vi "Flush Queue.vi"(8 "error in (no error)":errorcluster, 10 "Data Type":T12, 11 "Sift Client in":refnum<class "Sift Client.lvclass">) -> (0 "error out":errorcluster, 3 "Sift Client out":refnum<class "Sift Client.lvclass">)   [LabVIEW 2024, in "Sift Client.lvlib" / "Sift Client.lvclass"]
uses:
  Sift Client.lvclass
  Generate Sift Protos/SiftProxy_client/RPC Messages/sift_proxy_v1_ChannelDataType.ctl
  Generate Sift Protos/SiftProxy_client/RPC Messages/sift_proxy_v1_IngestDataStreamDoubleRequest.ctl
  Generate Sift Protos/SiftProxy_client/RPC Messages/google_protobuf_Timestamp.ctl
  Generate Sift Protos/SiftProxy_client/RPC Messages/sift_proxy_v1_IngestDataStreamStringRequest.ctl
  Generate Sift Protos/SiftProxy_client/RPC Messages/sift_proxy_v1_IngestDataStreamEnumRequest.ctl
  Generate Sift Protos/SiftProxy_client/RPC Messages/sift_proxy_v1_IngestDataStreamBytesRequest.ctl
  Generate Sift Protos/SiftProxy_client/RPC Messages/sift_proxy_v1_IngestDataStreamBoolRequest.ctl
  Generate Sift Protos/SiftProxy_client/RPC Messages/sift_proxy_v1_IngestDataStreamFloatRequest.ctl
  Generate Sift Protos/SiftProxy_client/RPC Messages/sift_proxy_v1_IngestDataStreamInt32Request.ctl
  Generate Sift Protos/SiftProxy_client/RPC Messages/sift_proxy_v1_IngestDataStreamUInt32Request.ctl
  Generate Sift Protos/SiftProxy_client/RPC Messages/sift_proxy_v1_IngestDataStreamInt64Request.ctl
  Generate Sift Protos/SiftProxy_client/RPC Messages/sift_proxy_v1_IngestDataStreamUInt64Request.ctl
  Sift Client.lvclass/Sift Client.ctl
  Generate Sift Protos/SiftProxy_client/SiftProxy_client.lvlib
panel:
  in  "sift_proxy_v1_IngestDataStreamUInt64Request":T1
  in  "sift_proxy_v1_IngestDataStreamInt64Request":T3
  in  "sift_proxy_v1_IngestDataStreamUInt32Request":T4
  in  "sift_proxy_v1_IngestDataStreamInt32Request":T5
  in  "sift_proxy_v1_IngestDataStreamFloatRequest":T6
  in  "sift_proxy_v1_IngestDataStreamBoolRequest":T7
  in  "sift_proxy_v1_IngestDataStreamBytesRequest":T8
  in  "sift_proxy_v1_IngestDataStreamEnumRequest":T9
  in  "sift_proxy_v1_IngestDataStreamStringRequest":T10
  in  "sift_proxy_v1_IngestDataStreamDoubleRequest":T11
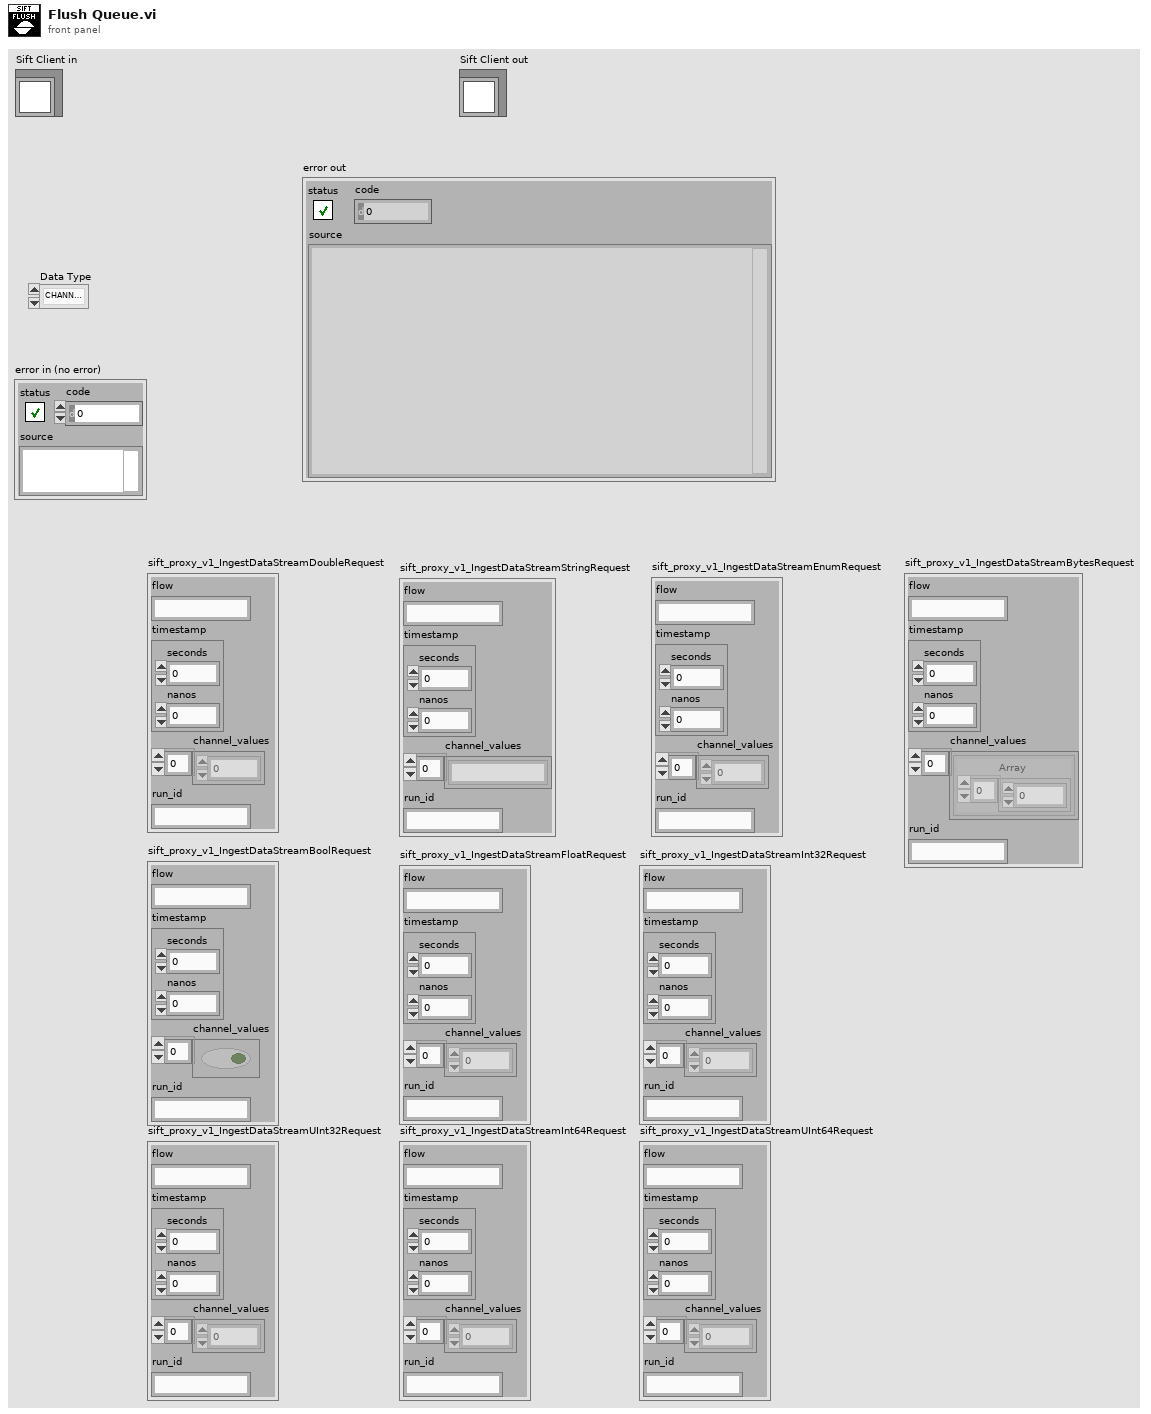
[diagram p1: front panel]
types:
  T1 = typedef "SiftProxy_client.lvlib/sift_proxy_v1_IngestDataStreamUInt64Request.ctl" = cluster{"flow":string, "timestamp":T2, "channel_values":u64[], "run_id":string}
  T2 = typedef "SiftProxy_client.lvlib/google_protobuf_Timestamp.ctl" = cluster{"seconds":i64, "nanos":i32}
  T3 = typedef "SiftProxy_client.lvlib/sift_proxy_v1_IngestDataStreamInt64Request.ctl" = cluster{"flow":string, "timestamp":T2, "channel_values":i64[], "run_id":string}
  T4 = typedef "SiftProxy_client.lvlib/sift_proxy_v1_IngestDataStreamUInt32Request.ctl" = cluster{"flow":string, "timestamp":T2, "channel_values":u32[], "run_id":string}
  T5 = typedef "SiftProxy_client.lvlib/sift_proxy_v1_IngestDataStreamInt32Request.ctl" = cluster{"flow":string, "timestamp":T2, "channel_values":i32[], "run_id":string}
  T6 = typedef "SiftProxy_client.lvlib/sift_proxy_v1_IngestDataStreamFloatRequest.ctl" = cluster{"flow":string, "timestamp":T2, "channel_values":sgl[], "run_id":string}
  T7 = typedef "SiftProxy_client.lvlib/sift_proxy_v1_IngestDataStreamBoolRequest.ctl" = cluster{"flow":string, "timestamp":T2, "channel_values":bool[], "run_id":string}
  T8 = typedef "SiftProxy_client.lvlib/sift_proxy_v1_IngestDataStreamBytesRequest.ctl" = cluster{"flow":string, "timestamp":T2, "channel_values":cluster{"Array":u8[]}[], "run_id":string}
  T9 = typedef "SiftProxy_client.lvlib/sift_proxy_v1_IngestDataStreamEnumRequest.ctl" = cluster{"flow":string, "timestamp":T2, "channel_values":u32[], "run_id":string}
  T10 = typedef "SiftProxy_client.lvlib/sift_proxy_v1_IngestDataStreamStringRequest.ctl" = cluster{"flow":string, "timestamp":T2, "channel_values":string[], "run_id":string}
  T11 = typedef "SiftProxy_client.lvlib/sift_proxy_v1_IngestDataStreamDoubleRequest.ctl" = cluster{"flow":string, "timestamp":T2, "channel_values":dbl[], "run_id":string}
  T12 = typedef "SiftProxy_client.lvlib/sift_proxy_v1_ChannelDataType.ctl" = enum32{"CHANNEL_DATA_TYPE_UNSPECIFIED", "CHANNEL_DATA_TYPE_DOUBLE", "CHANNEL_DATA_TYPE_STRING", "CHANNEL_DATA_TYPE_ENUM", "CHANNEL_DATA_TYPE_BIT_FIELD", "CHANNEL_DATA_TYPE_BOOL", "CHANNEL_DATA_TYPE_FLOAT", "CHANNEL_DATA_TYPE_INT_32", "CHANNEL_DATA_TYPE_UINT_32", "CHANNEL_DATA_TYPE_INT_64", "CHANNEL_DATA_TYPE_UINT_64"}
  T13 = typedef "Sift Client.lvlib/Double Sample.ctl" = cluster{"Values":dbl[], "Timestamp":T2, "Flow Name":string}
  T14 = typedef "grpc-lvsupport-release.lvlib/grpcId.ctl" = u64
  T15 = typedef "Sift Client.lvlib/String Sample.ctl" = cluster{"Values":string[], "Timestamp":T2, "Flow Name":string}
  T16 = typedef "Sift Client.lvlib/Enum Sample.ctl" = cluster{"Values":u32[], "Timestamp":T2, "Flow Name":string}
  T17 = typedef "Sift Client.lvlib/Bitfield Sample.ctl" = cluster{"Timestamp":T2, "Values":cluster{"Array":u8[]}[], "Flow Name":string}
  T18 = typedef "Sift Client.lvlib/Bool Sample.ctl" = cluster{"Values":bool[], "Timestamp":T2, "Flow Name":string}
  T19 = typedef "Sift Client.lvlib/Float Sample.ctl" = cluster{"Values":sgl[], "Timestamp":T2, "Flow Name":string}
  T20 = typedef "Sift Client.lvlib/Int32 Sample.ctl" = cluster{"Values":i32[], "Timestamp":T2, "Flow Name":string}
  T21 = typedef "Sift Client.lvlib/Uint32 Sample.ctl" = cluster{"Values":u32[], "Timestamp":T2, "Flow Name":string}
  T22 = typedef "Sift Client.lvlib/Int64 Sample.ctl" = cluster{"Values":i64[], "Timestamp":T2, "Flow Name":string}
  T23 = typedef "Sift Client.lvlib/Uint64 Sample.ctl" = cluster{"Values":u64[], "Timestamp":T2, "Flow Name":string}
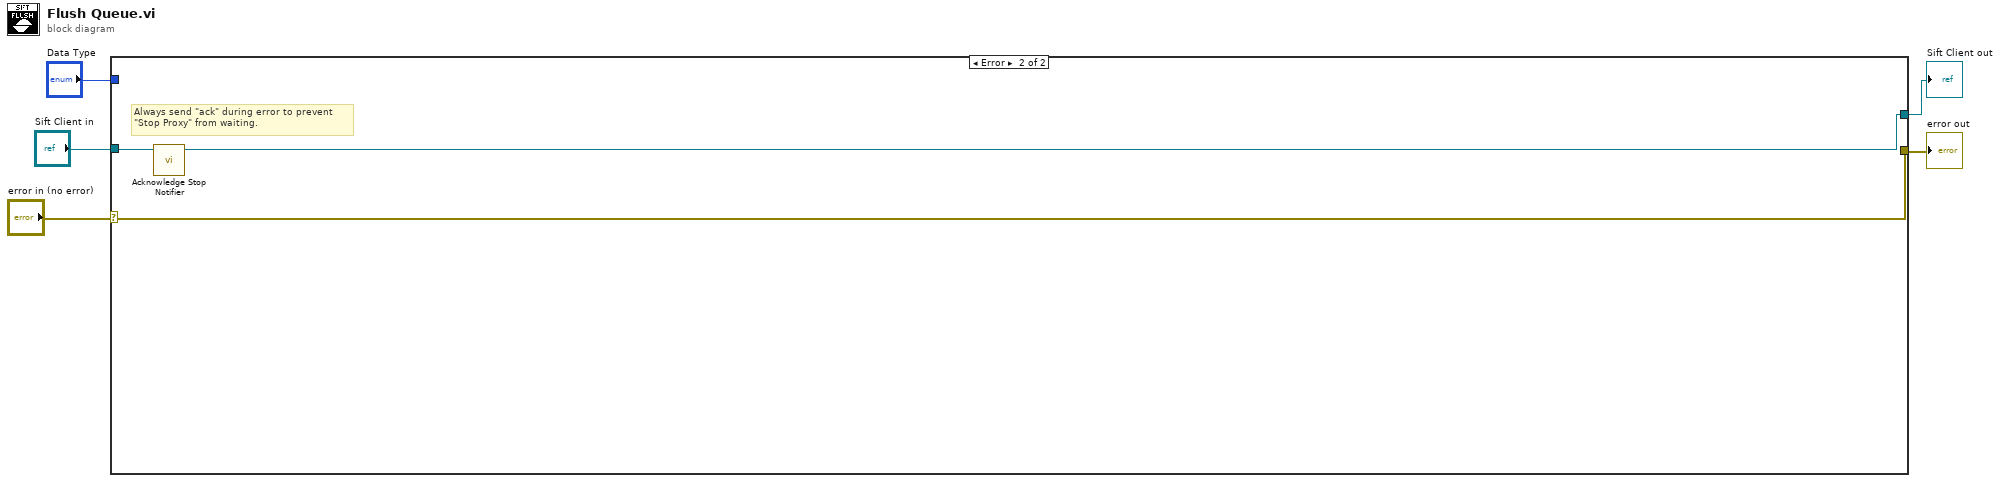
[diagram p0: block diagram]
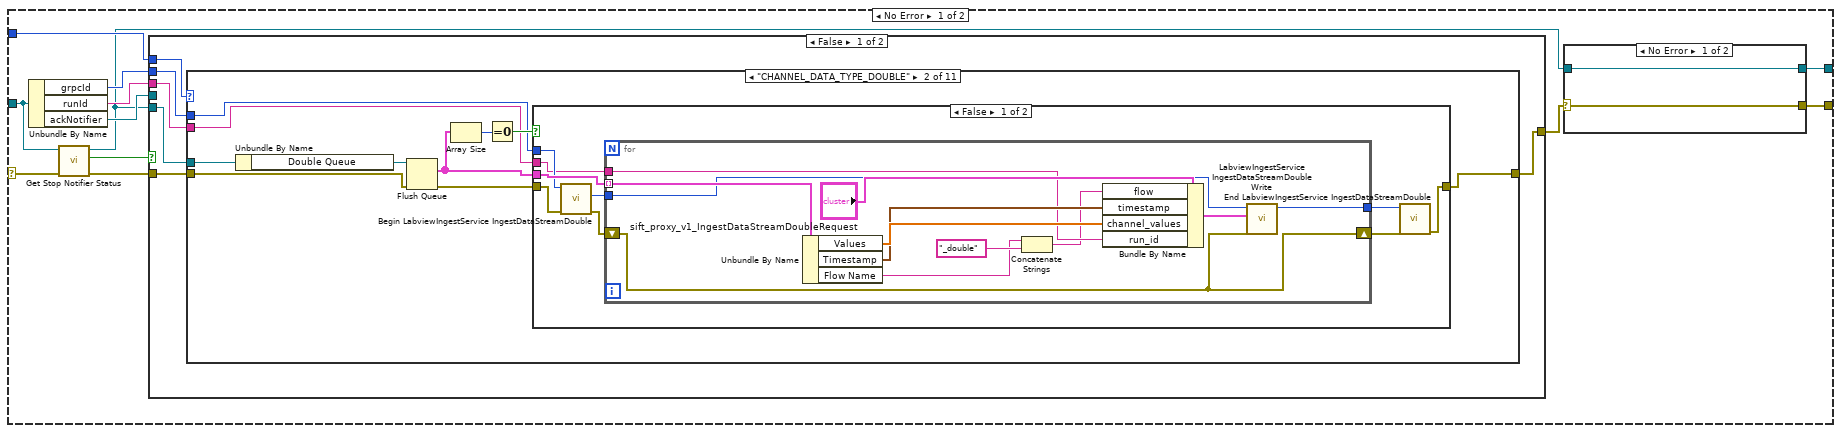
[diagram p2: hidden frame]
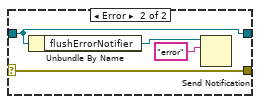
[diagram p3: hidden frame]
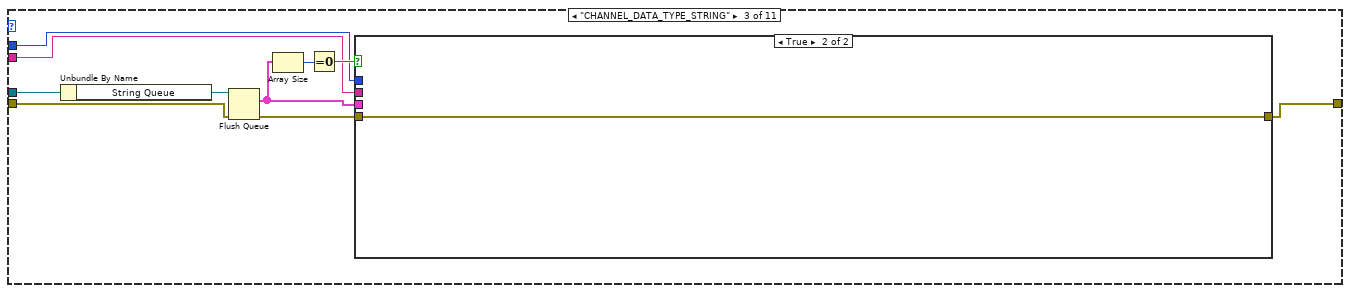
[diagram p6: hidden frame]
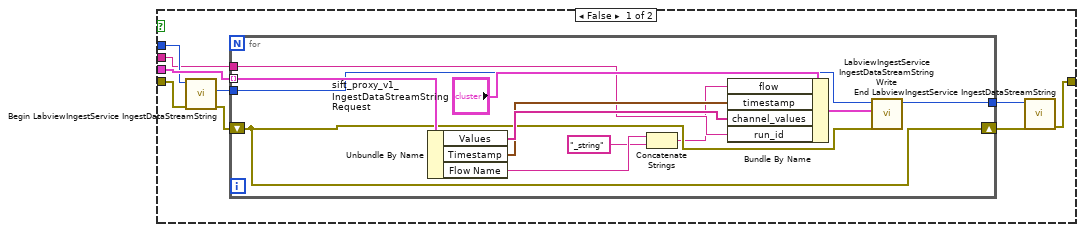
[diagram p7: hidden frame]
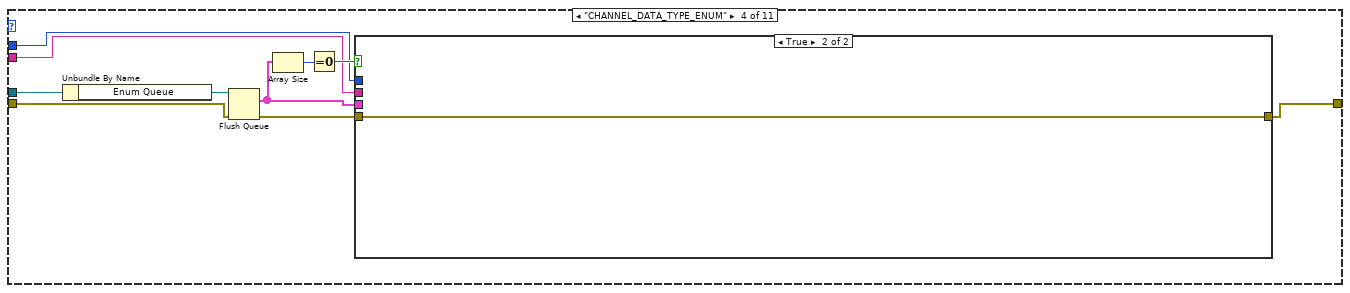
[diagram p8: hidden frame]
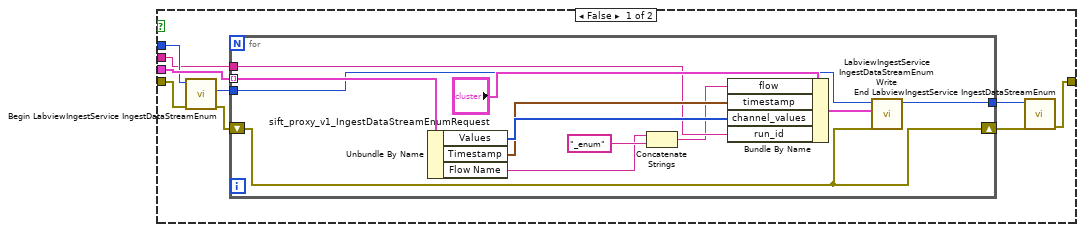
[diagram p9: hidden frame]
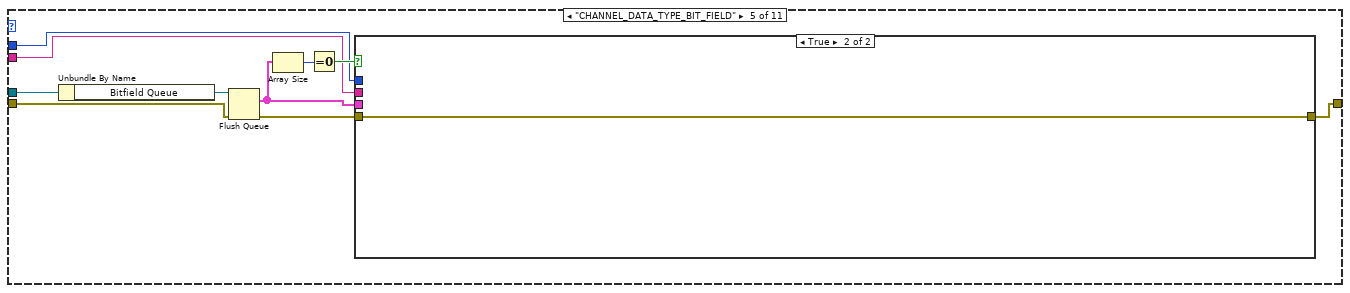
[diagram p10: hidden frame]
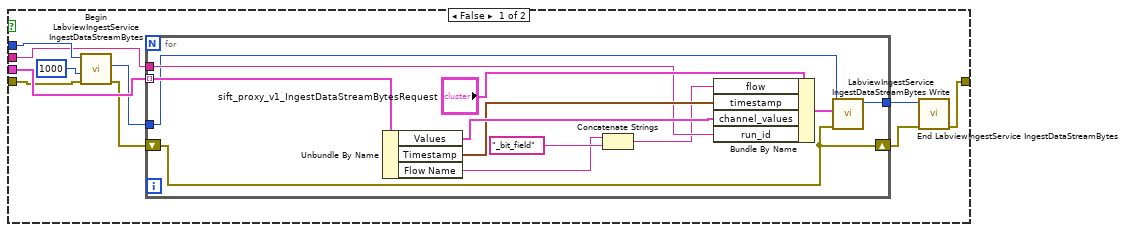
[diagram p11: hidden frame]
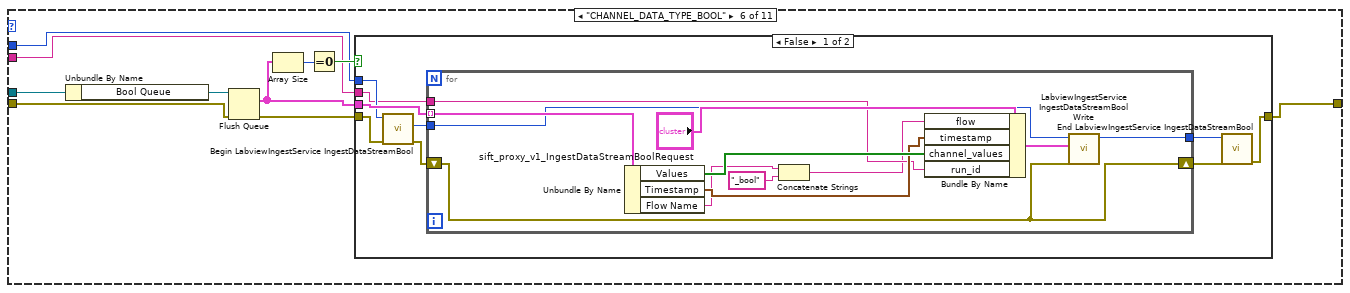
[diagram p12: hidden frame]
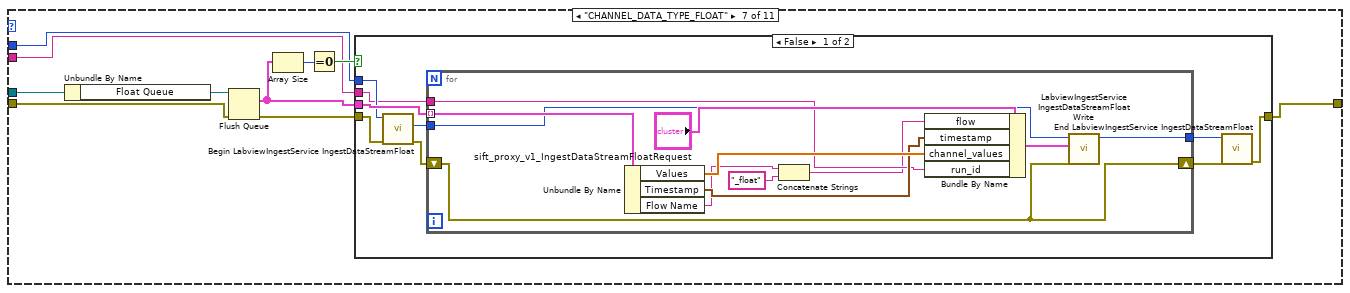
[diagram p14: hidden frame]
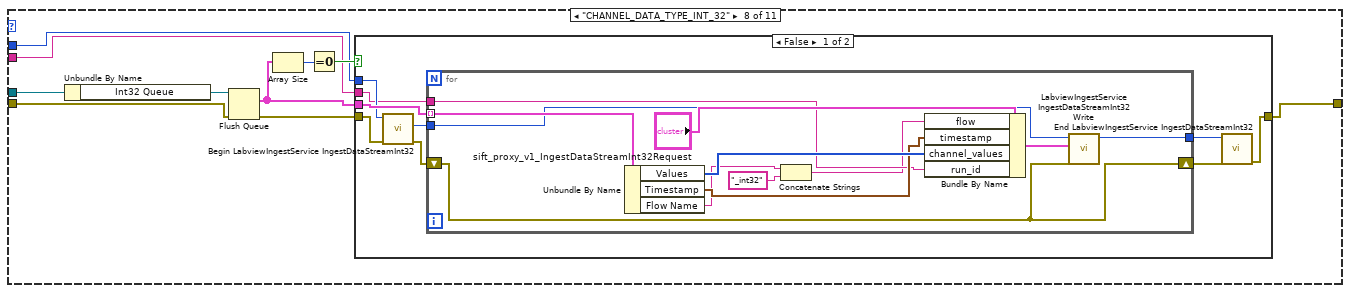
[diagram p16: hidden frame]
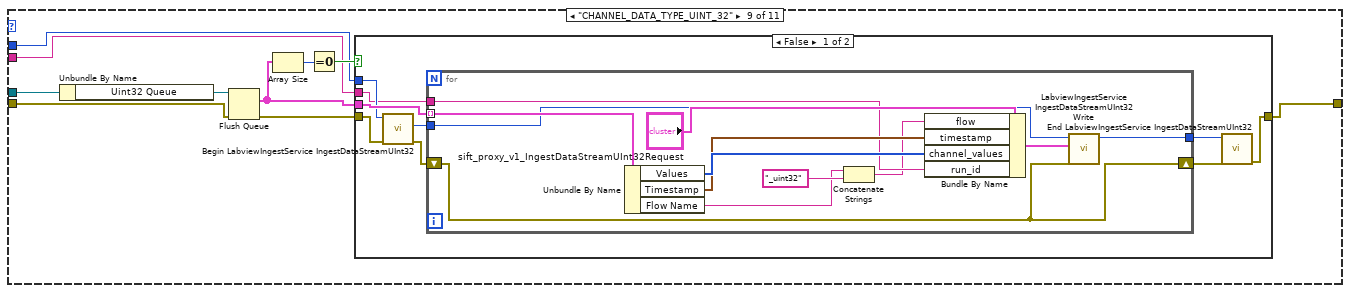
[diagram p18: hidden frame]
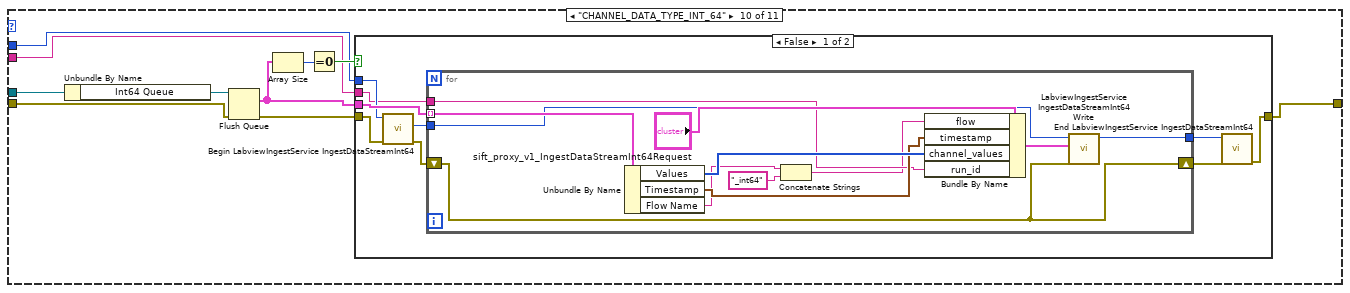
[diagram p20: hidden frame]
diagram:
  n1 = case shown="Error" "error in (no error)" {
    selector: "error in (no error)" -> [w12 w357]
    tunnel: [w8 w357] -> w4
    tunnel: [w6 w355] -> w2
    tunnel: "Sift Client in" -> [w13 w356]
    tunnel: "Data Type" -> [w17 _]
    frame No Error {
      n2 = Unbundle By Name(w13) -> ("grpcId"=w16:u64, "runId"=w15:string, "ackNotifier"=w14:refnum<notifier>)
      n3 = call-dynamic "Get Stop Notifier Status.vi"("error in (no error)"=w12, "Sift Client in"=w13) -> ("error out"=w11:errorcluster, "Fired"=w10:bool, "Sift Client out"=w7:refnum<class "Sift Client.lvclass">)  [unwired: 7 in]
      n4 = case shown="False" w10 {
        tunnel: w17 -> [w29 _]
        tunnel: w11 -> [w28 w354]
        tunnel: w7 -> [w27 w352]
        tunnel: w16 -> [w26 _]
        tunnel: w15 -> [w25 _]
        tunnel: [w24 w353] -> w9
        tunnel: w14 -> [_ _]
        frame False {
          n5 = case shown="\"CHANNEL_DATA_TYPE_DOUBLE\"" w29 {
            tunnel: w27 -> [_ w40 w72 w104 w136 w169 w201 w233 w265 w297 w329]
            tunnel: w28 -> [w30 w32 w64 w96 w128 w161 w193 w225 w257 w289 w321]
            tunnel: w26 -> [_ w35 w67 w99 w131 w164 w196 w228 w260 w292 w324]
            tunnel: w25 -> [_ w34 w66 w98 w130 w163 w195 w227 w259 w291 w323]
            tunnel: [w30 w33 w65 w97 w129 w162 w194 w226 w258 w290 w322] -> w24
            frame "CHANNEL_DATA_TYPE_UNSPECIFIED", Default {
            }
            frame "CHANNEL_DATA_TYPE_DOUBLE" {
              n6 = Unbundle By Name(w40) -> ("Double Queue"=w39:refnum<queue>)
              n7 = Flush Queue(queue=w39, error in (no error)=w32) -> (remaining elements=w36:T13[], error out=w31:errorcluster)  [unwired: 1 out]
              n8 = Array Size(array=w36) -> (size(s)=w38:i32)
              n9 = Equal To 0?(x=w38) -> (x = 0?=w37:bool)
              n10 = case shown="False" w37 {
                tunnel: w36 -> [w49 _]
                tunnel: w35 -> [w48 _]
                tunnel: w34 -> [w47 _]
                tunnel: w31 -> [w44 w62]
                tunnel: [w41 w62] -> w33
                frame False {
                  n11 = call "Begin LabviewIngestService IngestDataStreamDouble.vi"("error in"=w44, "gRPC ID"=w48) -> ("error out"=w43:errorcluster, "Call Id Out"=w46:T14)  [unwired: 7 in, 1 out]
                  n12 = for {
                    tunnel: w49 -> [w60] mode=indexing
                    tunnel: w47 -> [w57]
                    tunnel: w46 -> [w56]
                    tunnel: [w55] -> w45
                    shift-right: [w53] -> w42
                    shift-left: w43 -> [w53]
                    n13 = Unbundle By Name(w60) -> ("Values"=w59:dbl[], "Timestamp"=w58:T2, "Flow Name"=w51:string)
                    n14 = Concatenate Strings(w51, "_double") -> (w50:string)
                    n15 = Bundle By Name(cluster="sift_proxy_v1_IngestDataStreamDoubleRequest", "flow"=w50, "timestamp"=w58, "channel_values"=w59, "run_id"=w57) -> (w54:T11)
                    n16 = call "LabviewIngestService IngestDataStreamDouble Write.vi"("error in"=w53, "Request Data"=w54, "Call ID in"=w56) -> ("Call ID"=w55:T14)  [unwired: 6 in, 2 out]
                  }
                  n17 = call "End LabviewIngestService IngestDataStreamDouble.vi"("error in"=w42, "Call ID in"=w45) -> ("error out"=w41:errorcluster)  [unwired: 7 in, 2 out]
                }
                frame True {
                }
              }
            }
            frame "CHANNEL_DATA_TYPE_STRING" {
              n18 = Unbundle By Name(w72) -> ("String Queue"=w71:refnum<queue>)
              n19 = Flush Queue(queue=w71, error in (no error)=w64) -> (remaining elements=w68:T15[], error out=w63:errorcluster)  [unwired: 1 out]
              n20 = Array Size(array=w68) -> (size(s)=w70:i32)
              n21 = Equal To 0?(x=w70) -> (x = 0?=w69:bool)
              n22 = case shown="True" w69 {
                tunnel: w68 -> [w81 _]
                tunnel: w67 -> [w80 _]
                tunnel: w66 -> [w79 _]
                tunnel: w63 -> [w76 w94]
                tunnel: [w73 w94] -> w65
                frame False {
                  n23 = call "Begin LabviewIngestService IngestDataStreamString.vi"("error in"=w76, "gRPC ID"=w80) -> ("error out"=w75:errorcluster, "Call Id Out"=w78:T14)  [unwired: 7 in, 1 out]
                  n24 = for {
                    tunnel: w81 -> [w92] mode=indexing
                    tunnel: w79 -> [w89]
                    tunnel: w78 -> [w88]
                    tunnel: [w87] -> w77
                    shift-right: [w85] -> w74
                    shift-left: w75 -> [w85]
                    n25 = Unbundle By Name(w92) -> ("Values"=w91:string[], "Timestamp"=w90:T2, "Flow Name"=w84:string)
                    n26 = Concatenate Strings(w84, "_string") -> (w82:string)
                    n27 = Bundle By Name(cluster="sift_proxy_v1_IngestDataStreamStringRequest", "flow"=w82, "timestamp"=w90, "channel_values"=w91, "run_id"=w89) -> (w86:T10)
                    n28 = call "LabviewIngestService IngestDataStreamString Write.vi"("error in"=w85, "Request Data"=w86, "Call ID in"=w88) -> ("Call ID"=w87:T14)  [unwired: 6 in, 2 out]
                  }
                  n29 = call "End LabviewIngestService IngestDataStreamString.vi"("error in"=w74, "Call ID in"=w77) -> ("error out"=w73:errorcluster)  [unwired: 7 in, 2 out]
                }
                frame True {
                }
              }
            }
            frame "CHANNEL_DATA_TYPE_ENUM" {
              n30 = Unbundle By Name(w104) -> ("Enum Queue"=w103:refnum<queue>)
              n31 = Flush Queue(queue=w103, error in (no error)=w96) -> (remaining elements=w100:T16[], error out=w95:errorcluster)  [unwired: 1 out]
              n32 = Array Size(array=w100) -> (size(s)=w102:i32)
              n33 = Equal To 0?(x=w102) -> (x = 0?=w101:bool)
              n34 = case shown="True" w101 {
                tunnel: w100 -> [w113 _]
                tunnel: w99 -> [w112 _]
                tunnel: w98 -> [w111 _]
                tunnel: w95 -> [w108 w126]
                tunnel: [w105 w126] -> w97
                frame False {
                  n35 = call "Begin LabviewIngestService IngestDataStreamEnum.vi"("error in"=w108, "gRPC ID"=w112) -> ("error out"=w107:errorcluster, "Call Id Out"=w110:T14)  [unwired: 7 in, 1 out]
                  n36 = for {
                    tunnel: w113 -> [w124] mode=indexing
                    tunnel: w111 -> [w121]
                    tunnel: w110 -> [w120]
                    tunnel: [w119] -> w109
                    shift-right: [w117] -> w106
                    shift-left: w107 -> [w117]
                    n37 = Unbundle By Name(w124) -> ("Values"=w123:u32[], "Timestamp"=w122:T2, "Flow Name"=w115:string)
                    n38 = Concatenate Strings(w115, "_enum") -> (w114:string)
                    n39 = Bundle By Name(cluster="sift_proxy_v1_IngestDataStreamEnumRequest", "flow"=w114, "timestamp"=w122, "channel_values"=w123, "run_id"=w121) -> (w118:T9)
                    n40 = call "LabviewIngestService IngestDataStreamEnum Write.vi"("error in"=w117, "Request Data"=w118, "Call ID in"=w120) -> ("Call ID"=w119:T14)  [unwired: 6 in, 2 out]
                  }
                  n41 = call "End LabviewIngestService IngestDataStreamEnum.vi"("error in"=w106, "Call ID in"=w109) -> ("error out"=w105:errorcluster)  [unwired: 7 in, 2 out]
                }
                frame True {
                }
              }
            }
            frame "CHANNEL_DATA_TYPE_BIT_FIELD" {
              n42 = Unbundle By Name(w136) -> ("Bitfield Queue"=w135:refnum<queue>)
              n43 = Flush Queue(queue=w135, error in (no error)=w128) -> (remaining elements=w132:T17[], error out=w127:errorcluster)  [unwired: 1 out]
              n44 = Array Size(array=w132) -> (size(s)=w134:i32)
              n45 = Equal To 0?(x=w134) -> (x = 0?=w133:bool)
              n46 = case shown="True" w133 {
                tunnel: w132 -> [w146 _]
                tunnel: w131 -> [w145 _]
                tunnel: w130 -> [w144 _]
                tunnel: w127 -> [w141 w159]
                tunnel: [w138 w159] -> w129
                frame False {
                  n47 = call "Begin LabviewIngestService IngestDataStreamBytes.vi"("error in"=w141, "timeout (ms)"=1000, "gRPC ID"=w145) -> ("error out"=w140:errorcluster, "Call Id Out"=w143:T14)  [unwired: 6 in, 1 out]
                  n48 = for {
                    tunnel: w146 -> [w157] mode=indexing
                    tunnel: w144 -> [w154]
                    tunnel: w143 -> [w153]
                    tunnel: [w152] -> w142
                    shift-right: [w150] -> w139
                    shift-left: w140 -> [w150]
                    n49 = Unbundle By Name(w157) -> ("Values"=w156:cluster{"Array":u8[]}[], "Timestamp"=w155:T2, "Flow Name"=w148:string)
                    n50 = Concatenate Strings(w148, "_bit_field") -> (w147:string)
                    n51 = Bundle By Name(cluster="sift_proxy_v1_IngestDataStreamBytesRequest", "flow"=w147, "timestamp"=w155, "channel_values"=w156, "run_id"=w154) -> (w151:T8)
                    n52 = call "LabviewIngestService IngestDataStreamBytes Write.vi"("error in"=w150, "Request Data"=w151, "Call ID in"=w153) -> ("Call ID"=w152:T14)  [unwired: 6 in, 2 out]
                  }
                  n53 = call "End LabviewIngestService IngestDataStreamBytes.vi"("error in"=w139, "Call ID in"=w142) -> ("error out"=w138:errorcluster)  [unwired: 7 in, 2 out]
                }
                frame True {
                }
              }
            }
            frame "CHANNEL_DATA_TYPE_BOOL" {
              n54 = Unbundle By Name(w169) -> ("Bool Queue"=w168:refnum<queue>)
              n55 = Flush Queue(queue=w168, error in (no error)=w161) -> (remaining elements=w165:T18[], error out=w160:errorcluster)  [unwired: 1 out]
              n56 = Array Size(array=w165) -> (size(s)=w167:i32)
              n57 = Equal To 0?(x=w167) -> (x = 0?=w166:bool)
              n58 = case shown="False" w166 {
                tunnel: w165 -> [w178 _]
                tunnel: w164 -> [w177 _]
                tunnel: w163 -> [w176 _]
                tunnel: w160 -> [w173 w191]
                tunnel: [w170 w191] -> w162
                frame False {
                  n59 = call "Begin LabviewIngestService IngestDataStreamBool.vi"("error in"=w173, "gRPC ID"=w177) -> ("error out"=w172:errorcluster, "Call Id Out"=w175:T14)  [unwired: 7 in, 1 out]
                  n60 = for {
                    tunnel: w178 -> [w189] mode=indexing
                    tunnel: w176 -> [w186]
                    tunnel: w175 -> [w185]
                    tunnel: [w184] -> w174
                    shift-right: [w182] -> w171
                    shift-left: w172 -> [w182]
                    n61 = Unbundle By Name(w189) -> ("Values"=w188:bool[], "Timestamp"=w187:T2, "Flow Name"=w179:string)
                    n62 = Concatenate Strings(w179, "_bool") -> (w180:string)
                    n63 = Bundle By Name(cluster="sift_proxy_v1_IngestDataStreamBoolRequest", "flow"=w180, "timestamp"=w187, "channel_values"=w188, "run_id"=w186) -> (w183:T7)
                    n64 = call "LabviewIngestService IngestDataStreamBool Write.vi"("error in"=w182, "Request Data"=w183, "Call ID in"=w185) -> ("Call ID"=w184:T14)  [unwired: 6 in, 2 out]
                  }
                  n65 = call "End LabviewIngestService IngestDataStreamBool.vi"("error in"=w171, "Call ID in"=w174) -> ("error out"=w170:errorcluster)  [unwired: 7 in, 2 out]
                }
                frame True {
                }
              }
            }
            frame "CHANNEL_DATA_TYPE_FLOAT" {
              n66 = Unbundle By Name(w201) -> ("Float Queue"=w200:refnum<queue>)
              n67 = Flush Queue(queue=w200, error in (no error)=w193) -> (remaining elements=w197:T19[], error out=w192:errorcluster)  [unwired: 1 out]
              n68 = Array Size(array=w197) -> (size(s)=w199:i32)
              n69 = Equal To 0?(x=w199) -> (x = 0?=w198:bool)
              n70 = case shown="False" w198 {
                tunnel: w197 -> [w210 _]
                tunnel: w196 -> [w209 _]
                tunnel: w195 -> [w208 _]
                tunnel: w192 -> [w205 w223]
                tunnel: [w202 w223] -> w194
                frame False {
                  n71 = call "Begin LabviewIngestService IngestDataStreamFloat.vi"("error in"=w205, "gRPC ID"=w209) -> ("error out"=w204:errorcluster, "Call Id Out"=w207:T14)  [unwired: 7 in, 1 out]
                  n72 = for {
                    tunnel: w210 -> [w221] mode=indexing
                    tunnel: w208 -> [w218]
                    tunnel: w207 -> [w217]
                    tunnel: [w216] -> w206
                    shift-right: [w214] -> w203
                    shift-left: w204 -> [w214]
                    n73 = Unbundle By Name(w221) -> ("Values"=w220:sgl[], "Timestamp"=w219:T2, "Flow Name"=w212:string)
                    n74 = Concatenate Strings(w212, "_float") -> (w211:string)
                    n75 = Bundle By Name(cluster="sift_proxy_v1_IngestDataStreamFloatRequest", "flow"=w211, "timestamp"=w219, "channel_values"=w220, "run_id"=w218) -> (w215:T6)
                    n76 = call "LabviewIngestService IngestDataStreamFloat Write.vi"("error in"=w214, "Request Data"=w215, "Call ID in"=w217) -> ("Call ID"=w216:T14)  [unwired: 6 in, 2 out]
                  }
                  n77 = call "End LabviewIngestService IngestDataStreamFloat.vi"("error in"=w203, "Call ID in"=w206) -> ("error out"=w202:errorcluster)  [unwired: 7 in, 2 out]
                }
                frame True {
                }
              }
            }
            frame "CHANNEL_DATA_TYPE_INT_32" {
              n78 = Unbundle By Name(w233) -> ("Int32 Queue"=w232:refnum<queue>)
              n79 = Flush Queue(queue=w232, error in (no error)=w225) -> (remaining elements=w229:T20[], error out=w224:errorcluster)  [unwired: 1 out]
              n80 = Array Size(array=w229) -> (size(s)=w231:i32)
              n81 = Equal To 0?(x=w231) -> (x = 0?=w230:bool)
              n82 = case shown="False" w230 {
                tunnel: w229 -> [w242 _]
                tunnel: w228 -> [w241 _]
                tunnel: w227 -> [w240 _]
                tunnel: w224 -> [w237 w255]
                tunnel: [w234 w255] -> w226
                frame False {
                  n83 = call "Begin LabviewIngestService IngestDataStreamInt32.vi"("error in"=w237, "gRPC ID"=w241) -> ("error out"=w236:errorcluster, "Call Id Out"=w239:T14)  [unwired: 7 in, 1 out]
                  n84 = for {
                    tunnel: w242 -> [w253] mode=indexing
                    tunnel: w240 -> [w250]
                    tunnel: w239 -> [w249]
                    tunnel: [w248] -> w238
                    shift-right: [w246] -> w235
                    shift-left: w236 -> [w246]
                    n85 = Unbundle By Name(w253) -> ("Values"=w252:i32[], "Timestamp"=w251:T2, "Flow Name"=w244:string)
                    n86 = Concatenate Strings(w244, "_int32") -> (w243:string)
                    n87 = Bundle By Name(cluster="sift_proxy_v1_IngestDataStreamInt32Request", "flow"=w243, "timestamp"=w251, "channel_values"=w252, "run_id"=w250) -> (w247:T5)
                    n88 = call "LabviewIngestService IngestDataStreamInt32 Write.vi"("error in"=w246, "Request Data"=w247, "Call ID in"=w249) -> ("Call ID"=w248:T14)  [unwired: 6 in, 2 out]
                  }
                  n89 = call "End LabviewIngestService IngestDataStreamInt32.vi"("error in"=w235, "Call ID in"=w238) -> ("error out"=w234:errorcluster)  [unwired: 7 in, 2 out]
                }
                frame True {
                }
              }
            }
            frame "CHANNEL_DATA_TYPE_UINT_32" {
              n90 = Unbundle By Name(w265) -> ("Uint32 Queue"=w264:refnum<queue>)
              n91 = Flush Queue(queue=w264, error in (no error)=w257) -> (remaining elements=w261:T21[], error out=w256:errorcluster)  [unwired: 1 out]
              n92 = Array Size(array=w261) -> (size(s)=w263:i32)
              n93 = Equal To 0?(x=w263) -> (x = 0?=w262:bool)
              n94 = case shown="False" w262 {
                tunnel: w261 -> [w274 _]
                tunnel: w260 -> [w273 _]
                tunnel: w259 -> [w272 _]
                tunnel: w256 -> [w269 w287]
                tunnel: [w266 w287] -> w258
                frame False {
                  n95 = call "Begin LabviewIngestService IngestDataStreamUInt32.vi"("error in"=w269, "gRPC ID"=w273) -> ("error out"=w268:errorcluster, "Call Id Out"=w271:T14)  [unwired: 7 in, 1 out]
                  n96 = for {
                    tunnel: w274 -> [w285] mode=indexing
                    tunnel: w272 -> [w282]
                    tunnel: w271 -> [w281]
                    tunnel: [w280] -> w270
                    shift-right: [w278] -> w267
                    shift-left: w268 -> [w278]
                    n97 = Unbundle By Name(w285) -> ("Values"=w284:u32[], "Timestamp"=w283:T2, "Flow Name"=w276:string)
                    n98 = Concatenate Strings(w276, "_uint32") -> (w275:string)
                    n99 = Bundle By Name(cluster="sift_proxy_v1_IngestDataStreamUInt32Request", "flow"=w275, "timestamp"=w283, "channel_values"=w284, "run_id"=w282) -> (w279:T4)
                    n100 = call "LabviewIngestService IngestDataStreamUInt32 Write.vi"("error in"=w278, "Request Data"=w279, "Call ID in"=w281) -> ("Call ID"=w280:T14)  [unwired: 6 in, 2 out]
                  }
                  n101 = call "End LabviewIngestService IngestDataStreamUInt32.vi"("error in"=w267, "Call ID in"=w270) -> ("error out"=w266:errorcluster)  [unwired: 7 in, 2 out]
                }
                frame True {
                }
              }
            }
            frame "CHANNEL_DATA_TYPE_INT_64" {
              n102 = Unbundle By Name(w297) -> ("Int64 Queue"=w296:refnum<queue>)
              n103 = Flush Queue(queue=w296, error in (no error)=w289) -> (remaining elements=w293:T22[], error out=w288:errorcluster)  [unwired: 1 out]
              n104 = Array Size(array=w293) -> (size(s)=w295:i32)
              n105 = Equal To 0?(x=w295) -> (x = 0?=w294:bool)
              n106 = case shown="False" w294 {
                tunnel: w293 -> [w306 _]
                tunnel: w292 -> [w305 _]
                tunnel: w291 -> [w304 _]
                tunnel: w288 -> [w301 w319]
                tunnel: [w298 w319] -> w290
                frame False {
                  n107 = call "Begin LabviewIngestService IngestDataStreamInt64.vi"("error in"=w301, "gRPC ID"=w305) -> ("error out"=w300:errorcluster, "Call Id Out"=w303:T14)  [unwired: 7 in, 1 out]
                  n108 = for {
                    tunnel: w306 -> [w317] mode=indexing
                    tunnel: w304 -> [w314]
                    tunnel: w303 -> [w313]
                    tunnel: [w312] -> w302
                    shift-right: [w310] -> w299
                    shift-left: w300 -> [w310]
                    n109 = Unbundle By Name(w317) -> ("Values"=w316:i64[], "Timestamp"=w315:T2, "Flow Name"=w308:string)
                    n110 = Concatenate Strings(w308, "_int64") -> (w307:string)
                    n111 = Bundle By Name(cluster="sift_proxy_v1_IngestDataStreamInt64Request", "flow"=w307, "timestamp"=w315, "channel_values"=w316, "run_id"=w314) -> (w311:T3)
                    n112 = call "LabviewIngestService IngestDataStreamInt64 Write.vi"("error in"=w310, "Request Data"=w311, "Call ID in"=w313) -> ("Call ID"=w312:T14)  [unwired: 6 in, 2 out]
                  }
                  n113 = call "End LabviewIngestService IngestDataStreamInt64.vi"("error in"=w299, "Call ID in"=w302) -> ("error out"=w298:errorcluster)  [unwired: 7 in, 2 out]
                }
                frame True {
                }
              }
            }
            frame "CHANNEL_DATA_TYPE_UINT_64" {
              n114 = Unbundle By Name(w329) -> ("Uint64 Queue"=w328:refnum<queue>)
              n115 = Flush Queue(queue=w328, error in (no error)=w321) -> (remaining elements=w325:T23[], error out=w320:errorcluster)  [unwired: 1 out]
              n116 = Array Size(array=w325) -> (size(s)=w327:i32)
              n117 = Equal To 0?(x=w327) -> (x = 0?=w326:bool)
              n118 = case shown="False" w326 {
                tunnel: w325 -> [w338 _]
                tunnel: w324 -> [w337 _]
                tunnel: w323 -> [w336 _]
                tunnel: w320 -> [w333 w351]
                tunnel: [w330 w351] -> w322
                frame False {
                  n119 = call "Begin LabviewIngestService IngestDataStreamUInt64.vi"("error in"=w333, "gRPC ID"=w337) -> ("error out"=w332:errorcluster, "Call Id Out"=w335:T14)  [unwired: 7 in, 1 out]
                  n120 = for {
                    tunnel: w338 -> [w349] mode=indexing
                    tunnel: w336 -> [w346]
                    tunnel: w335 -> [w345]
                    tunnel: [w344] -> w334
                    shift-right: [w342] -> w331
                    shift-left: w332 -> [w342]
                    n121 = Unbundle By Name(w349) -> ("Values"=w348:u64[], "Timestamp"=w347:T2, "Flow Name"=w340:string)
                    n122 = Concatenate Strings(w340, "_uint64") -> (w339:string)
                    n123 = Bundle By Name(cluster="sift_proxy_v1_IngestDataStreamUInt64Request", "flow"=w339, "timestamp"=w347, "channel_values"=w348, "run_id"=w346) -> (w343:T1)
                    n124 = call "LabviewIngestService IngestDataStreamUInt64 Write.vi"("error in"=w342, "Request Data"=w343, "Call ID in"=w345) -> ("Call ID"=w344:T14)  [unwired: 6 in, 2 out]
                  }
                  n125 = call "End LabviewIngestService IngestDataStreamUInt64.vi"("error in"=w331, "Call ID in"=w334) -> ("error out"=w330:errorcluster)  [unwired: 7 in, 2 out]
                }
                frame True {
                }
              }
            }
          }
        }
        frame True {
          n126 = call-dynamic "Acknowledge Stop Notifier.vi"("error in (no error)"=w354, "Sift Client in"=w352) -> ("error out"=w353:errorcluster)  [unwired: 8 in, 1 out]
        }
      }
      n127 = case shown="No Error" w9 {
        selector: w9 -> [w18 w21]
        tunnel: w7 -> [w19 w20]
        tunnel: [w18 w21] -> w8
        tunnel: [w19 w20] -> w6
        frame No Error {
        }
        frame Error {
          n128 = Unbundle By Name(w20) -> ("flushErrorNotifier"=w23:refnum<notifier>)
          n129 = Send Notification(notification="error", notifier=w23) -> ()  [unwired: 1 in, 2 out]
        }
      }
    }
    frame Error {
      # "Always send \"ack\" during error to prevent \n\"Stop Proxy\" from waiting."
      n130 = call-dynamic "Acknowledge Stop Notifier.vi"("Sift Client in"=w356) -> ("Sift Client out"=w355:refnum<class "Sift Client.lvclass">)  [unwired: 9 in, 1 out]
    }
  }
  "error out" <- w4
  "Sift Client out" <- w2
